vi "Convert_I16toDBL.vi"(6 "Input Range (mV)":u32=10000, 7 "DC Offset (mV)":i32, 8 "Offset":i16, 9 "Resolution":i32=-32768, 10 "Interger Signal":i32[](array[numeric])) -> (2 "Data in Volts":dbl[](array[numeric]) format="%.2f")   [LabVIEW 2011]
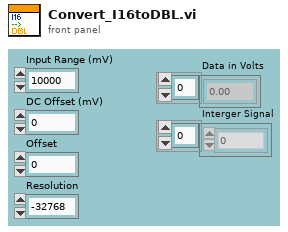
[diagram p1: front panel]
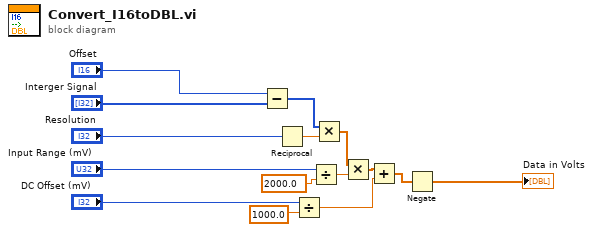
[diagram p0: block diagram]
diagram:
  n1 = Subtract(x="Offset", y="Interger Signal") -> (x-y=w15:i32[])
  n2 = Reciprocal(x="Resolution") -> (1/x=w3:dbl)
  n3 = Divide(x="DC Offset (mV)", y=1000.0) -> (x/y=w9:dbl)
  n4 = Divide(x="Input Range (mV)", y=2000.0) -> (x/y=w10:dbl)
  n5 = Multiply(x=w15, y=w3) -> (x*y=w11:dbl[])
  n6 = Multiply(x=w11, y=w10) -> (x*y=w13:dbl[])
  n7 = Add(x=w13, y=w9) -> (x+y=w2:dbl[])
  n8 = Negate(x=w2) -> (-x=→"Data in Volts":dbl[])
